vi "Export dialog.vi"(8 "error in (no error)":errorcluster, 10 "Available options":T2={"Clipboard"=TRUE, "dat"=TRUE, "iso"=FALSE, "Origin"=FALSE, "Excel"=FALSE}) -> (0 "error out":errorcluster, 2 "Canceled":bool, 3 "Option":T1(ring))   [LabVIEW 2019]
doc: "Displays a dialog window asking user for an export type"
uses:
  <vilib>/Utility/miscctls.llb/LVPointTypeDef.ctl
panel:
  in  "Buttons":T3
  # "Choose export type"
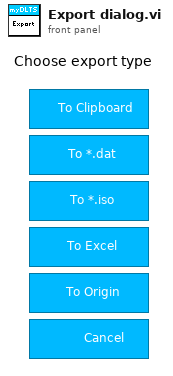
[diagram p1: front panel]
types:
  T1 = enum16{"Canceled", "Clipboard", "Dat", "Iso", "Origin", "Excel"}
  T2 = cluster{"Clipboard":bool, "dat":bool, "iso":bool, "Origin":bool, "Excel":bool}
  T3 = cluster{"Clipboard":bool, "dat":bool, "iso":bool, "Excel":bool, "Origin":bool, "Cancel":bool}
  T4 = typedef "LVPointTypeDef.ctl" = cluster{"Horizontal":i16, "Vertical":i16}
  T5 = typedef "LVRectTypeDef.ctl" = cluster{"Left":i16, "Top":i16, "Right":i16, "Bottom":i16}
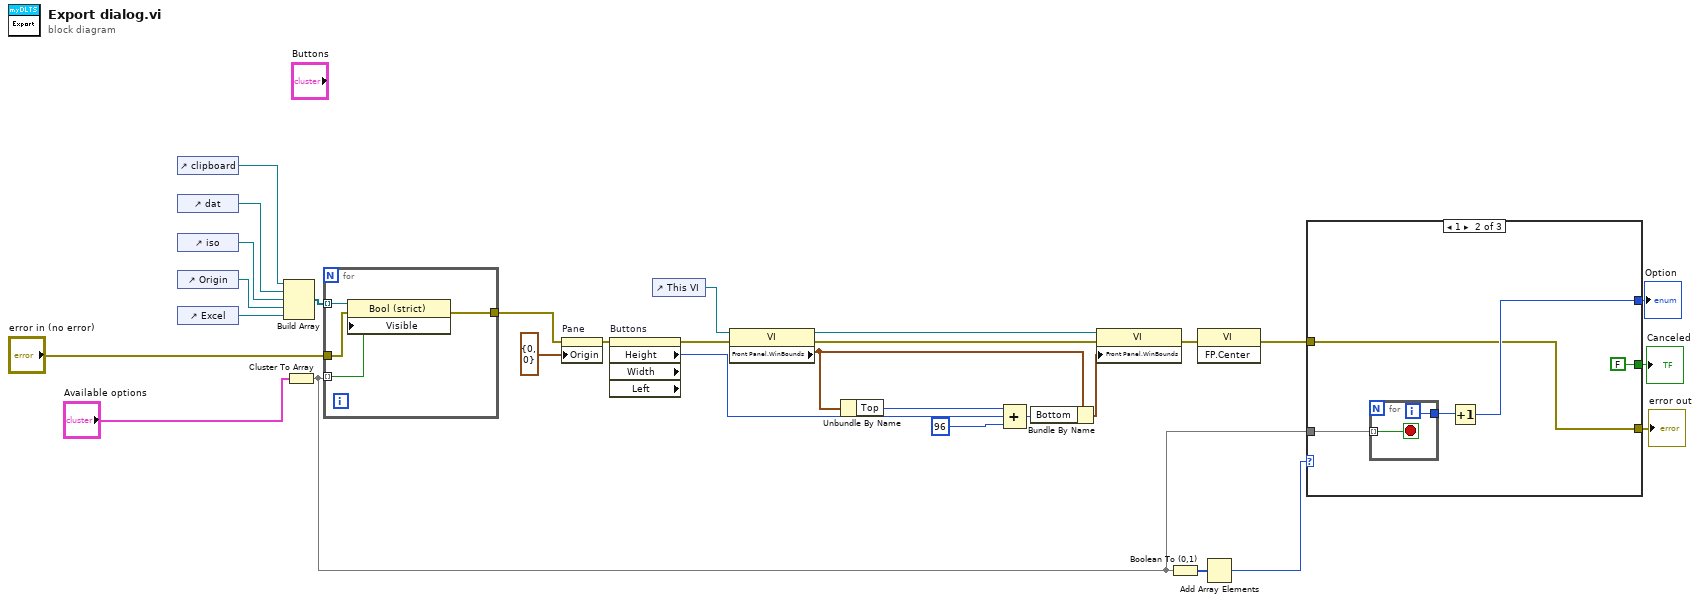
[diagram p0: block diagram]
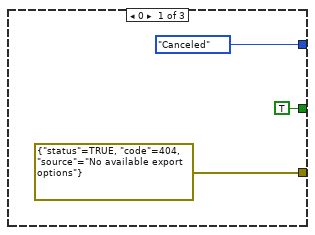
[diagram p2: hidden frame]
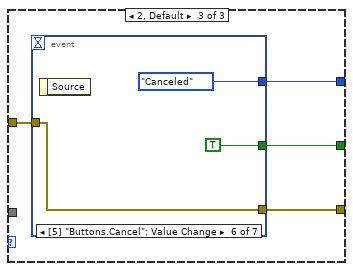
[diagram p3: hidden frame]
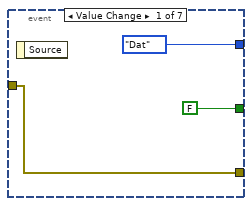
[diagram p4: hidden frame]
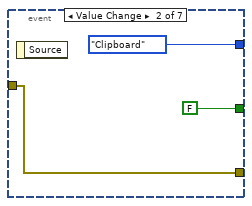
[diagram p5: hidden frame]
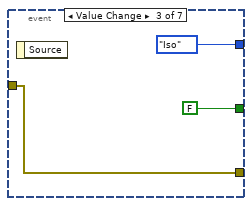
[diagram p6: hidden frame]
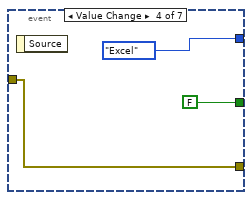
[diagram p7: hidden frame]
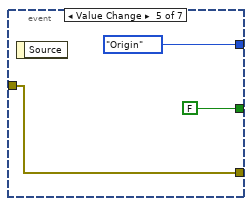
[diagram p8: hidden frame]
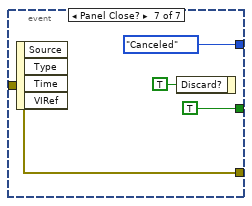
[diagram p9: hidden frame]
diagram:
  n1 = control-ref of="clipboard"() -> (w1:refnum<vi>)
  n2 = control-ref of="dat"() -> (w28:refnum<vi>)
  n3 = control-ref of="iso"() -> (w27:refnum<vi>)
  n4 = control-ref of="Origin"() -> (w26:refnum<vi>)
  n5 = control-ref of="Excel"() -> (w25:refnum<vi>)
  n6 = Build Array(w1, w28, w27, w26, w25) -> (w23:refnum<vi>[])
  n7 = Cluster To Array(cluster="Available options") -> (array=w2:bool[])
  n8 = for {
    tunnel: w23 -> [w33] mode=indexing
    tunnel: w2 -> [w32] mode=indexing
    tunnel: [w31] -> w22
    tunnel: "error in (no error)" -> [w30]
    n9 = property class="Bool (strict)"(reference=w33, error in=w30, "Visible"=w32) -> (error out=w31:errorcluster)  [unwired: 1 out]
  }
  n10 = property on="Pane" class="Pane"(error in=w22, "Origin"=T4 {"Horizontal"=0, "Vertical"=0}) -> (error out=w21:errorcluster)  [unwired: 1 in, 1 out]
  n11 = property on="Buttons" class="Clust (strict)" props=["Height", "Width", "Left"](error in=w21) -> (error out=w19:errorcluster, "Height"=w13:u32)  [unwired: 1 in, 3 out]
  n12 = control-ref of="This VI"() -> (w20:refnum<vi>)
  n13 = property class="VI"(reference=w20, error in=w19) -> (reference out=w17:refnum<vi>, error out=w18:errorcluster, "Front Panel.WinBounds"=w15:T5)
  n14 = Unbundle By Name(w15) -> ("Top"=w14:i16)
  n15 = Compound Arithmetic op=ADD(w14, w13, u32 96 ("y")) -> (w9:u32)
  n16 = Bundle By Name(cluster=w15, "Bottom"=w9) -> (w16:T5)
  n17 = property class="VI"(reference=w17, error in=w18, "Front Panel.WinBounds"=w16) -> (error out=w11:errorcluster)  [unwired: 1 out]
  n18 = Boolean To (0,1)(Boolean=w2) -> (0, 1=w4:i16[])
  n19 = invoke class="VI" method="FP.Center"(error in=w11) -> (error out=w10:errorcluster)  [unwired: 2 in, 2 out]
  n20 = Add Array Elements(numeric array=w4) -> (sum=w3:i16)
  n21 = case shown="1" w3 {
    tunnel: w10 -> [_ w37 w47]
    tunnel: [T1."Canceled" ("Option") w39 w46] -> w8
    tunnel: [errorcluster {"status"=TRUE, "code"=404, "source"="No available export options"} ("error out") w37 w45] -> w6
    tunnel: [TRUE ("Canceled") FALSE ("Canceled") w44] -> w5
    tunnel: w2 -> [_ w41 _]
    frame 0 {
    }
    frame 1 {
      n22 = for {
        tunnel: w41 -> [w43] mode=indexing
        tunnel: [w42] -> w40
        i -> [w42]
        stop <- w43 stop-if-true
      }
      n23 = Increment(x=w40) -> (x+1=w39:i32)
    }
    frame 2, Default {
      n24 = event shown="[5] \"Buttons.Cancel\": Value Change" {
        selector: _ -> [_ _ _ _ _ _ _]
        dyn-events: _ -> [_ _ _ _ _ _ _]
        timeout: _ -> [_ _ _ _ _ _ _]
        tunnel: w47 -> [w50 w53 w56 w59 w62 w65 w69]
        tunnel: [T1."Dat" ("Option") T1."Clipboard" ("Option") T1."Iso" ("Option") T1."Excel" ("Option") T1."Origin" ("Option") T1."Canceled" ("Option") T1."Canceled" ("Option")] -> w46
        tunnel: [w50 w53 w56 w59 w62 w65 w69] -> w45
        tunnel: [FALSE ("Canceled") FALSE ("Canceled") FALSE ("Canceled") FALSE ("Canceled") FALSE ("Canceled") TRUE ("Canceled") TRUE ("Canceled")] -> w44
        event "Buttons.dat": Value Change {
          n25 = event-data() -> ()  [unwired: 1 in, 1 out]
        }
        event "Buttons.Clipboard": Value Change {
          n26 = event-data() -> ()  [unwired: 1 in, 1 out]
        }
        event "Buttons.iso": Value Change {
          n27 = event-data() -> ()  [unwired: 1 in, 1 out]
        }
        event "Buttons.Excel": Value Change {
          n28 = event-data() -> ()  [unwired: 1 in, 1 out]
        }
        event "Buttons.Origin": Value Change {
          n29 = event-data() -> ()  [unwired: 1 in, 1 out]
        }
        event "Buttons.Cancel": Value Change {
          n30 = event-data() -> ()  [unwired: 1 in, 1 out]
        }
        event Panel Close? {
          n31 = event-data() -> ()  [unwired: 1 in, 4 out]
          n32 = event-data("Discard?"=TRUE) -> ()  [unwired: 1 in, 1 out]
        }
      }
    }
  }
  "Option" <- w8
  "error out" <- w6
  "Canceled" <- w5
